vi "Developer Error - Unhandled Case.vi"(8 "error in":errorcluster, 11 "VI Ref (calling VI)":refnum<vi>) -> (0 "error out":errorcluster)   [LabVIEW 2015, in "Utility.lvlib"]
uses:
  Utility.lvlib
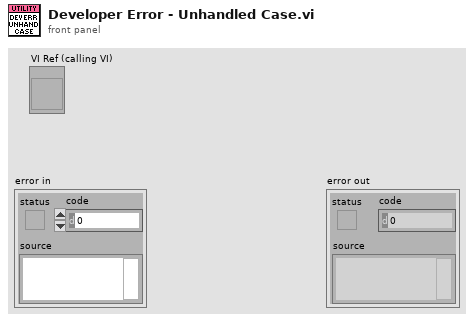
[diagram p1: front panel]
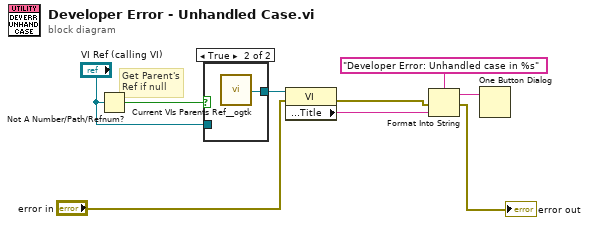
[diagram p0: block diagram]
diagram:
  # "Get Parent's\nRef if null"
  n1 = Not A Number/Path/Refnum?(number/path/refnum="VI Ref (calling VI)") -> (NaN/Path/Refnum?=w8:bool)
  n2 = case shown="True" w8 {
    tunnel: [w10 w11] -> w7
    tunnel: "VI Ref (calling VI)" -> [w10 _]
    frame False {
    }
    frame True {
      n3 = call <userlib>:"Current VIs Parents Ref__ogtk.vi"() -> ("Calling VI's Reference"=w11:refnum<vi>)  [unwired: 2 in]
    }
  }
  n4 = property class="VI"(reference=w7, error in="error in") -> (error out=w2:errorcluster, "Front Panel.Title"=w5:string)  [unwired: 1 out]
  n5 = Format Into String(format string="Developer Error: Unhandled case in %s", error in=w2, w5) -> (resulting string=w4:string, error out=→"error out":errorcluster)  [unwired: 1 in]
  n6 = One Button Dialog(message=w4) -> ()  [unwired: 1 in, 1 out]
